vi "SENS_MULT_PORT_SEL.vi"(0 "VISA IN":refnum<visa-resource-name>, 1 "ID":i32, 2 "Logical Port":i32, 3 "Physical Port":string, 5 "error in":errorcluster, 7 "Channel":i32) -> (14 "VISA Out":refnum<visa-resource-name>, 19 "error out":errorcluster)   [LabVIEW 2018, in "PNA-X.lvlib"]
doc: "SENSe<cnum>:MULTiplexer<id>:PORT<logi>SELect <phys> \n(Write-Only) Sets and returns a port mapping for a single port. If this command creates a conflict with \nan existing port, the PNA will resolve the conflict. \nNote: This command is currently not supported for the Z5623AK44. \nParameters \n<cnum> Channel number of the measurement. If unspecified, value is set to 1. \n<id> Id of the external test set. If unspecified, Id is assumed to be 1. Must be \npreviously set by the SENSe:MULT:TYPE command. \n<logi> Integer - Logical port number. \n<string> String - Physical port number. \nExamples SENS:MULT1:PORT3:SEL \"4\" 'sets logical port 3 to physical port \n4. \nReturn Type String \nDefault Not Applicable \nSENSe:MULTiplexer<id>:STATe <bool> \n1784\n\n(Read-Write) Enables and disables (ON/OFF) the port mapping and control line output of the \nspecified test set. \nIf the specified test set is not connected or not ON, then setting State ON will report an error. All other \nproperties can be set when the test set is not connected. \nWhen this command is set to ON, then the display of the test set status bar (SENS:MULT:DISP) is \nalso set to ON. \nParameters \n<id> Id of the external test set. If unspecified, Id is assumed to be 1. Must be \npreviously set by the SENSe:MULT:TYPE command. \n<bool> ON(1) Enables test set control. \nOFF (0) Disables test set control. \nExamples SENS:MULT1:STAT 1 \nsense2:multiplexer2:state on \nQuery Syntax SENSe<cnum>:MULTiplexer<id>:STATe? \nReturn Type Boolean \nDefault OFF (0)"
uses:
  PNA-X.lvlib
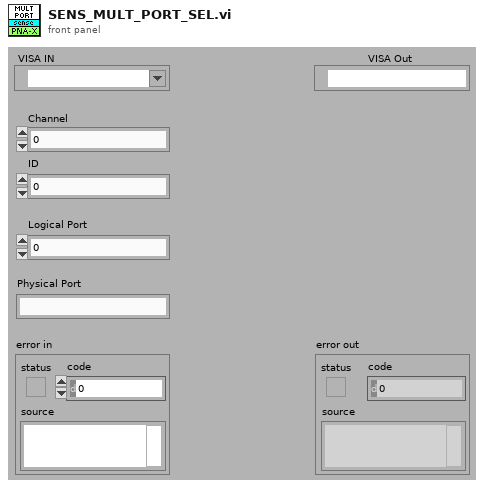
[diagram p1: front panel]
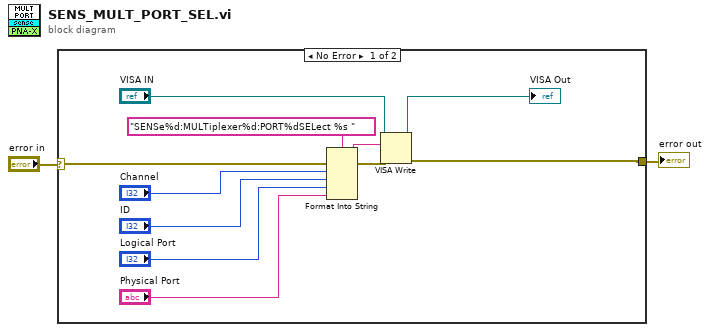
[diagram p0: block diagram]
diagram:
  n1 = case shown="No Error" "error in" {
    selector: "error in" -> [w13 w14]
    tunnel: [w8 w14] -> w1
    frame No Error {
      n2 = Format Into String(format string="SENSe%d:MULTiplexer%d:PORT%dSELect %s " ("Cmdline"), error in=w13, "Channel", "ID", "Logical Port", "Physical Port") -> (resulting string=w11:string, error out=w12:errorcluster)  [unwired: 1 in]
      n3 = VISA Write(VISA resource name="VISA IN", write buffer=w11, error in (no error)=w12) -> (VISA resource name out=→"VISA Out":refnum<visa-resource-name>, error out=w8:errorcluster)  [unwired: 1 out]
    }
    frame Error {
    }
  }
  "error out" <- w1
